vi "Read_Refresh_Token.vi"(8 "error in (no error)":errorcluster, 11 "Asana in":refnum<class "Asana.lvclass">) -> (0 "error out":errorcluster, 2 "Refresh Token":string, 3 "Asana out":refnum<class "Asana.lvclass">)   [LabVIEW 2016, in "Asana.lvclass"]
uses:
  Asana.lvclass
  Asana.lvclass/Asana.ctl
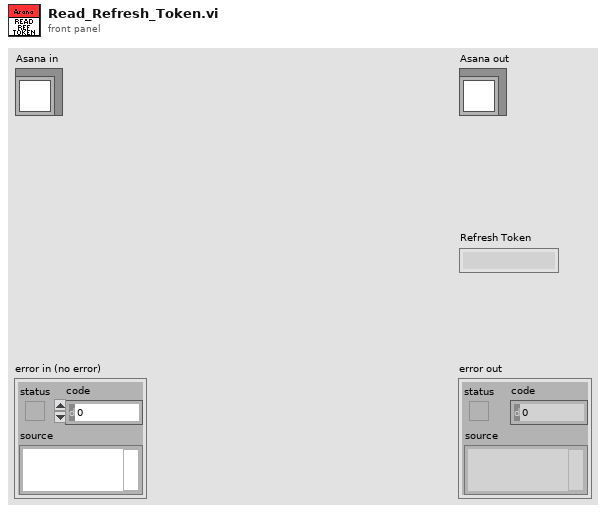
[diagram p1: front panel]
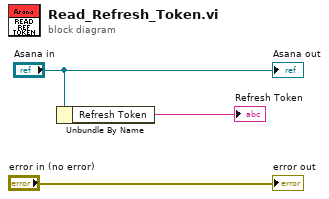
[diagram p0: block diagram]
diagram:
  n1 = Unbundle By Name("Asana in") -> ("Refresh Token"=→"Refresh Token":string)
  "error out" <- "error in (no error)"
  "Asana out" <- "Asana in"
